vi "getArrayNotZeroIdx.vi"(11 "Array":dbl[](array[numeric])) -> (3 "Index Array":i32[](array[numeric]))   [LabVIEW 2016]
doc: "Get the non-zero index array."
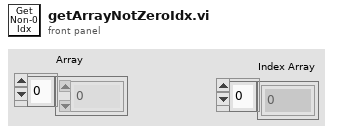
[diagram p1: front panel]
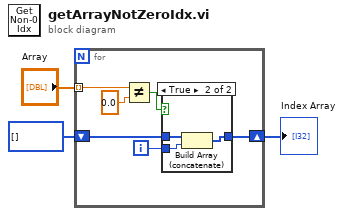
[diagram p0: block diagram]
diagram:
  n1 = for {
    tunnel: "Array" -> [w8] mode=indexing
    shift-right: [w4] -> w1
    shift-left: i32[] [] -> [w5]
    i -> [w6]
    n2 = Not Equal?(x=w8, y=0.0) -> (x != y?=w9:bool)
    n3 = case shown="True" w9 {
      tunnel: w6 -> [_ w13]
      tunnel: w5 -> [w10 w12]
      tunnel: [w10 w11] -> w4
      frame False {
      }
      frame True {
        n4 = Build Array (concatenate)(w12, w13) -> (w11:i32[])
      }
    }
  }
  "Index Array" <- w1
